vi "温度测量.vi"() -> ()   [LabVIEW 2018]
panel:
  out "波形图表":dbl(graph)
  out "最小值":dbl
  out "最大值":dbl
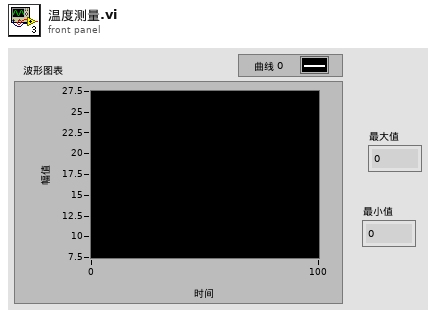
[diagram p1: front panel]
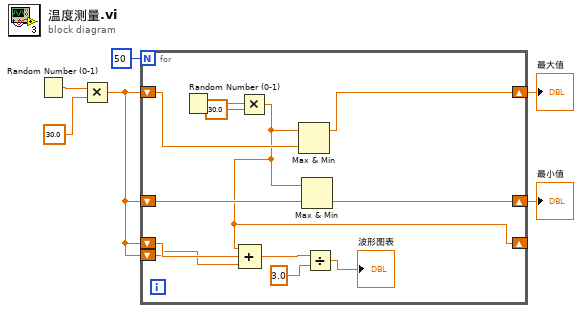
[diagram p0: block diagram]
diagram:
  n1 = Random Number (0-1)() -> (number: 0 to 1=w5:dbl)
  n2 = Multiply(x=w5, y=30.0) -> (x*y=w1:dbl)
  n3 = for {
    N: 50 -> [_]
    shift-right: [w15] -> w3
    shift-left: w1 -> [w16]
    shift-right: [w13] -> w2
    shift-left: w1 -> [w14]
    shift-right: [w10] -> _
    shift-left: w1 -> [w9]
    shift-left: w1 -> [w8]
    n4 = Random Number (0-1)() -> (number: 0 to 1=w17:dbl)
    n5 = Multiply(x=w17, y=30.0) -> (x*y=w10:dbl)
    n6 = Compound Arithmetic op=ADD(w10, w9, w8) -> (w11:dbl)
    n7 = Max & Min(x=w10, y=w16) -> (max(x,y)=w15:dbl)  [unwired: 1 out]
    n8 = Max & Min(x=w10, y=w14) -> (min(x,y)=w13:dbl)  [unwired: 1 out]
    n9 = Divide(x=w11, y=3.0) -> (x/y=→"波形图表":dbl)
  }
  "最大值" <- w3
  "最小值" <- w2
